vi "Send-message.vi"(4 "SenderID":i32, 6 "Sender":string, 8 "error in (no error)":errorcluster, 9 "Receivers":string[](array[string]), 10 "Message":refnum<class "Message.lvclass">, 11 "Server in":T1) -> (0 "error out":errorcluster, 3 "Server out":T1)   [LabVIEW 2013, in "SLMServer.lvlib" / "SLMServer.lvclass"]
uses:
  SLMServer.lvclass
  Object-reference.ctl
  SA-SLMAPI/Sources/Message.lvclass
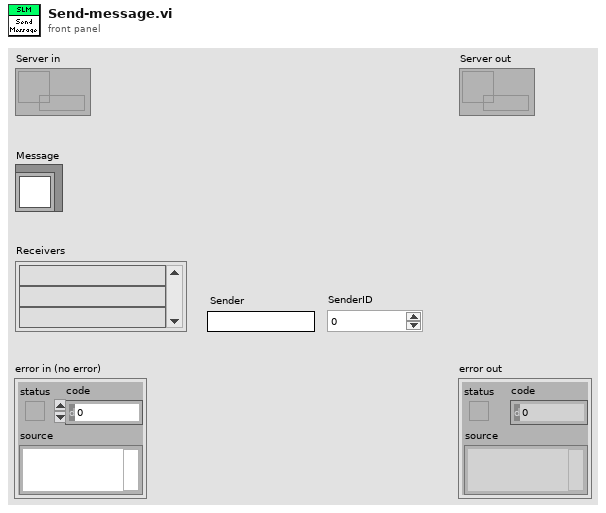
[diagram p1: front panel]
types:
  T1 = typedef "SLMServer.lvlib/SLMServer.lvclass/Object-reference.ctl" = refnum<data-value>
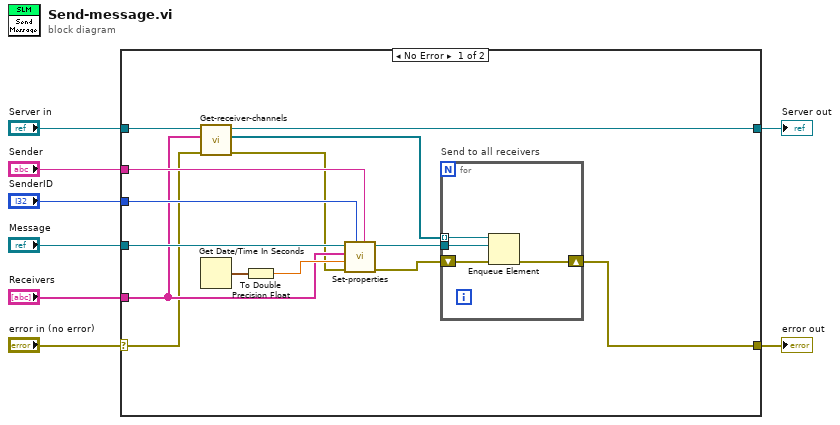
[diagram p0: block diagram]
diagram:
  n1 = case shown="No Error" "error in (no error)" {
    selector: "error in (no error)" -> [w12 w28]
    tunnel: [w21 w28] -> w7
    tunnel: [w9 w27] -> w5
    tunnel: "Server in" -> [w16 w27]
    tunnel: "Message" -> [w22 _]
    tunnel: "Receivers" -> [w15 _]
    tunnel: "SenderID" -> [w18 _]
    tunnel: "Sender" -> [w17 _]
    frame No Error {
      n2 = call "Get-receiver-channels.vi"("error in (no error)"=w12, "Receivers"=w15, "ModComm in"=w16) -> ("error out"=w11:errorcluster, "Receiver channels"=w10:refnum<queue>[], "ModComm out"=w9:T1)  [unwired: 6 in]
      n3 = Get Date/Time In Seconds() -> (seconds since 1Jan1904=w20:timestamp)
      n4 = To Double Precision Float(number=w20) -> (double precision float=w19:dbl)
      n5 = call-dynamic "Set-properties.vi"("Sender type"=w17, "Sender ID"=w18, "error in (no error)"=w11, "Send time"=w19, "Receivers"=w15, "Message in"=w22) -> ("error out"=w13:errorcluster, "Message out"=w14:refnum<class "Message.lvclass">)  [unwired: 4 in]
      n6 = for "Send to all receivers" {
        tunnel: w14 -> [w25]
        tunnel: w10 -> [w23] mode=indexing
        shift-right: [w26] -> w21
        shift-left: w13 -> [w24]
        n7 = Enqueue Element(queue=w23, element=w25, error in (no error)=w24) -> (error out=w26:errorcluster)  [unwired: 1 in, 2 out]
      }
    }
    frame Error {
    }
  }
  "error out" <- w7
  "Server out" <- w5
